vi "Identities.vi"(8 "error in (no error)":errorcluster, 11 "API in":refnum<class "API.lvclass">) -> (0 "error out":errorcluster, 2 "Identities":refnum<class "Identity.lvclass">[](array[class]), 3 "API out":refnum<class "API.lvclass">)   [LabVIEW 2020, in "Volatus.lvlib" / "API.lvclass"]
uses:
  API.lvclass
  Identity/Identity.lvclass
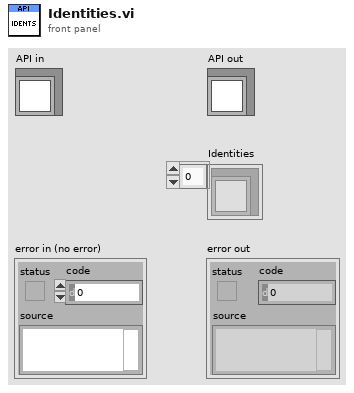
[diagram p1: front panel]
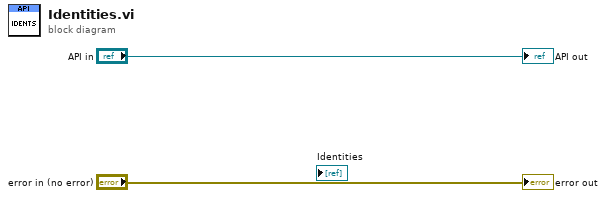
[diagram p0: block diagram]
diagram:
  "error out" <- "error in (no error)"
  "API out" <- "API in"
